vi "Run.vi"(8 "error in (no error)":errorcluster caption="entrée d'erreur (pas d'erreur)", 9 "y":string[][](array[string]), 10 "x":string[][](array[string]), 11 "Auc.lvclass":refnum<class "Auc.lvclass">) -> (0 "error out":errorcluster caption="sortie d'erreur", 2 "Score":string, 3 "Auc.lvclass":refnum<class "Auc.lvclass">)   [LabVIEW 2020, in "Auc.lvclass"]
doc: "Returns :\n\n- auc : float"
uses:
  Auc.lvclass
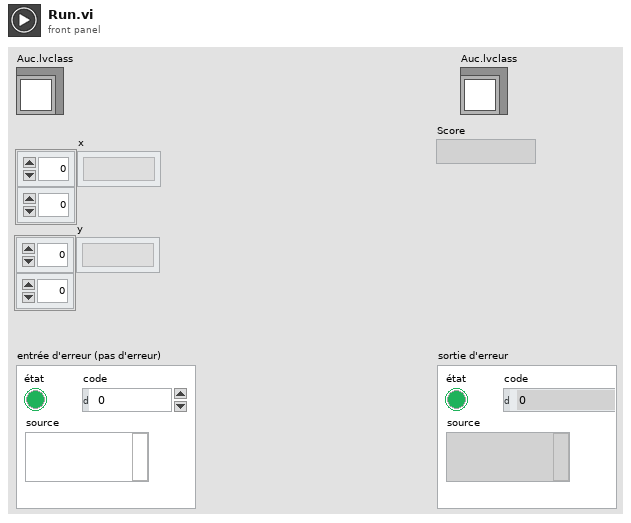
[diagram p1: front panel]
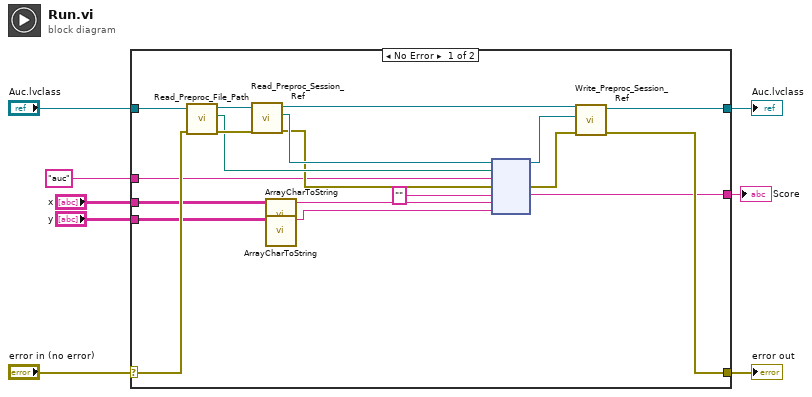
[diagram p0: block diagram]
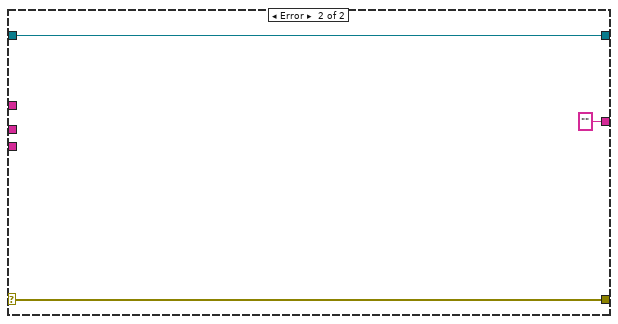
[diagram p2: hidden frame]
diagram:
  n1 = case shown="No Error" "error in (no error)" {
    selector: "error in (no error)" -> [w16 w30]
    tunnel: [w17 w30] -> w7
    tunnel: [w14 w29] -> w5
    tunnel: "Auc.lvclass" -> [w18 w29]
    tunnel: "auc" -> [w15 _]
    tunnel: "x" -> [w12 _]
    tunnel: "y" -> [w11 _]
    tunnel: [w13 ""] -> w1
    frame No Error {
      n2 = call-dynamic "Read_Preproc_File_Path.vi"("error in (no error)"=w16, "Python in"=w18) -> ("error out"=w26:errorcluster, "File_Path"=w25:path, "Python out"=w27:refnum<class "Auc.lvclass">)  [unwired: 7 in]
      n3 = call-dynamic "Read_Preproc_Session_Ref.vi"("error in (no error)"=w26, "Python in"=w27) -> ("error out"=w23:errorcluster, "Session_ref"=w24:refnum<k35>, "Python out"=w22:refnum<class "Auc.lvclass">)  [unwired: 7 in]
      n4 = call "ArrayCharToString.vi"("TAB"=w12) -> ("Instruction"=w10:string)  [unwired: 10 in]
      n5 = call "ArrayCharToString.vi"("TAB"=w11) -> ("Instruction"=w9:string)  [unwired: 10 in]
      n6 = node(w24, w25, w15, w23, "", w10, w9) -> (w20:refnum<k35>, w21:errorcluster, w13:string)  [unwired: 2 in, 2 out]
      n7 = call-dynamic "Write_Preproc_Session_Ref.vi"("error in (no error)"=w21, "Session_ref"=w20, "Python in"=w22) -> ("error out"=w17:errorcluster, "Python out"=w14:refnum<class "Auc.lvclass">)  [unwired: 7 in]
    }
    frame Error {
    }
  }
  "error out" <- w7
  "Auc.lvclass" <- w5
  "Score" <- w1
